vi "LogResult.vi"(5 "Mode":T1, 8 "Test Result":errorcluster, 10 "Test Artifact":T2 format="%x", 11 "VI Path":path) -> ()   [LabVIEW 2013]
uses:
  <vilib>/Heliosphere Research LLC/Advanced Plotting Toolkit/typedefs/PlotID.ctl
  ModeType.ctl
  OutputDirectory.vi
  <vilib>/Heliosphere Research LLC/Advanced Plotting Toolkit/Advanced Plotting Toolkit.lvlib
panel:
  out "Log To Disk":bool
  out "Status Out":string
  out "Picture":picture
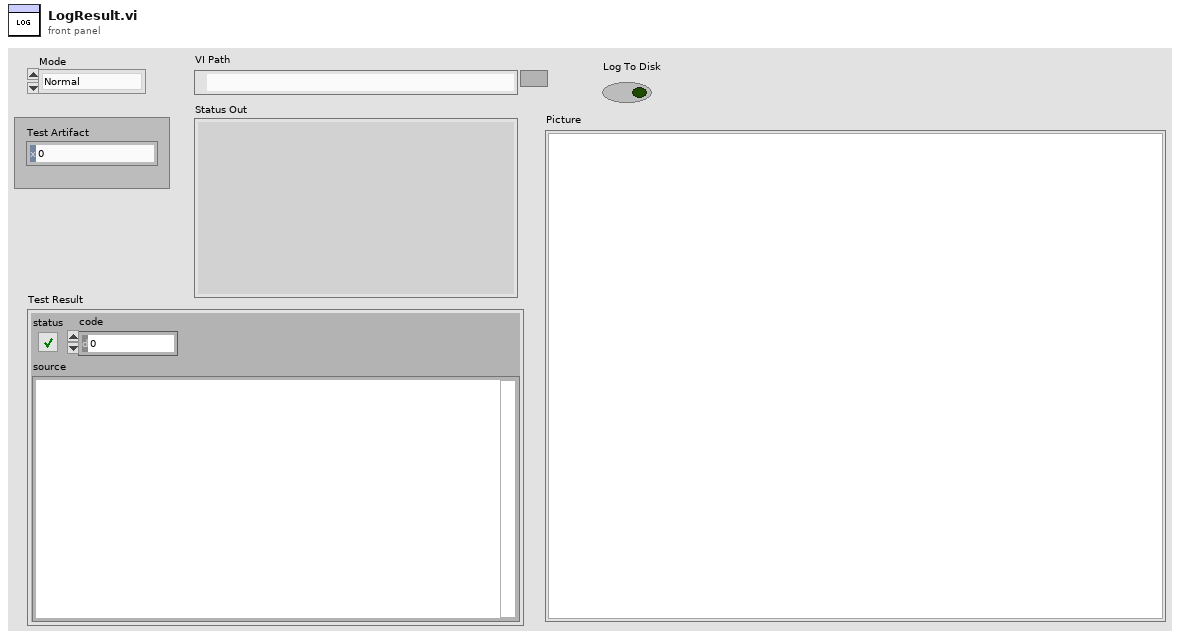
[diagram p1: front panel]
types:
  T1 = typedef "ModeType.ctl" = enum16{"Normal", "Expected Failure", "Skipped", "Broken"}
  T2 = typedef "Advanced Plotting Toolkit.lvlib/PlotID.ctl" = i32
  T3 = enum16{"open", "replace", "create", "open or create", "replace or create", "replace or create with confirmation"}
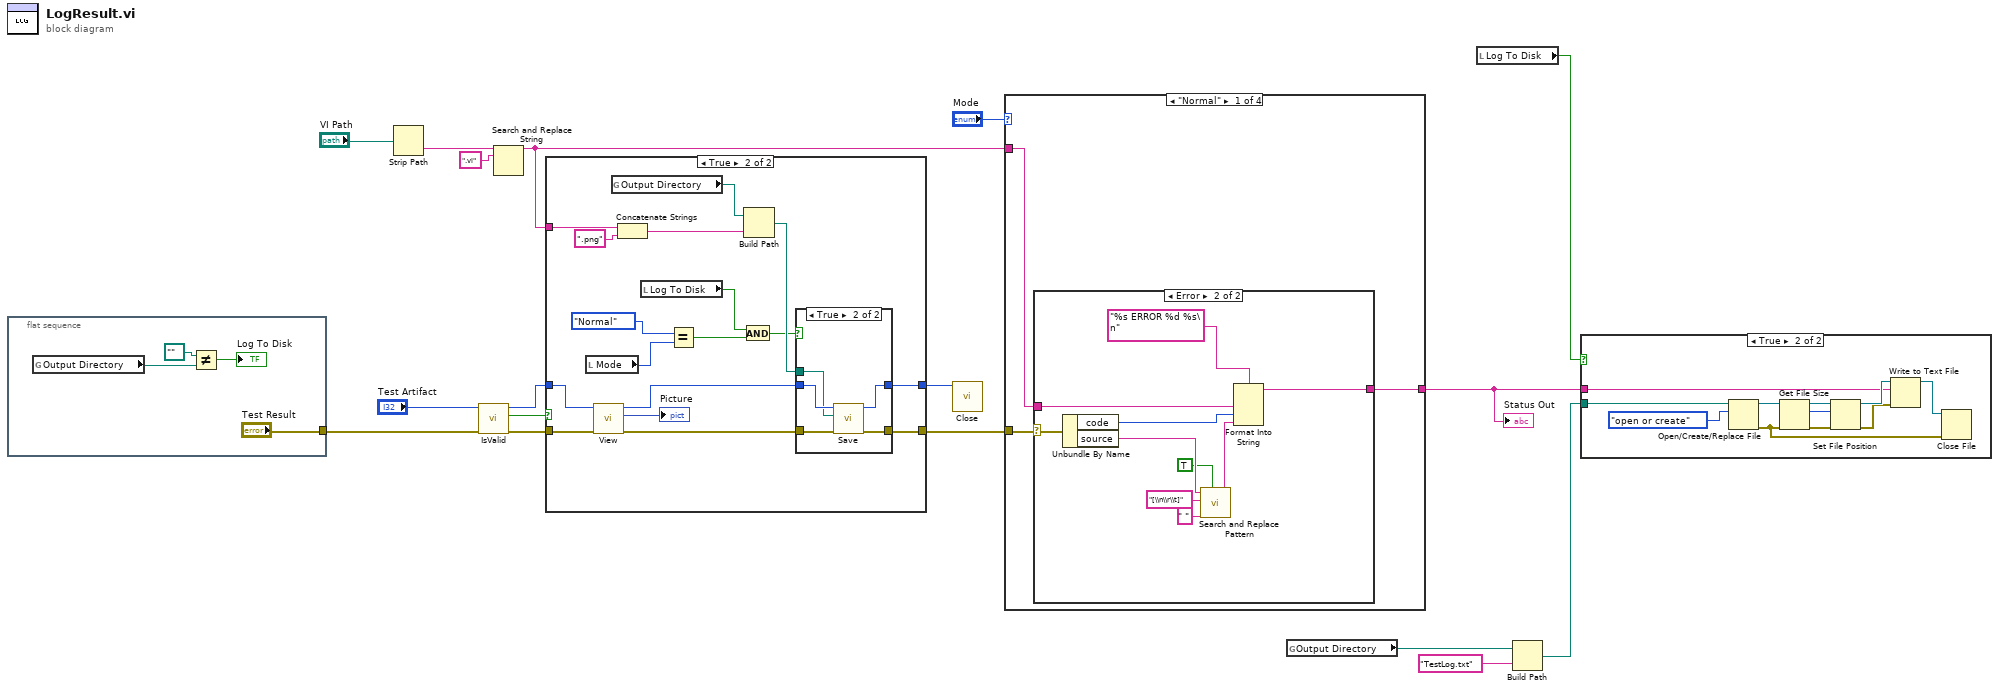
[diagram p0: block diagram]
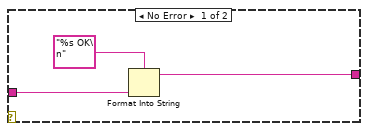
[diagram p2: hidden frame]
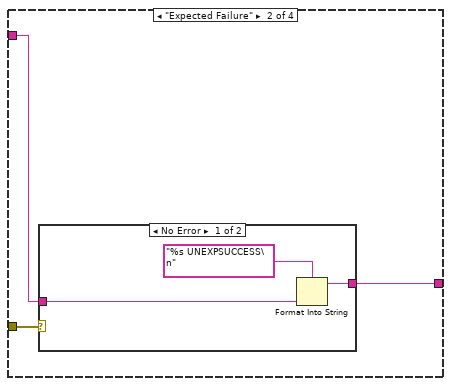
[diagram p3: hidden frame]
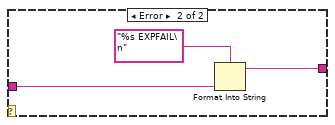
[diagram p4: hidden frame]
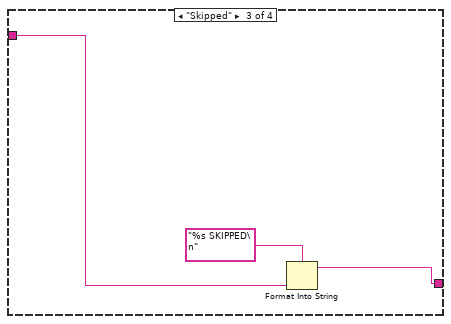
[diagram p5: hidden frame]
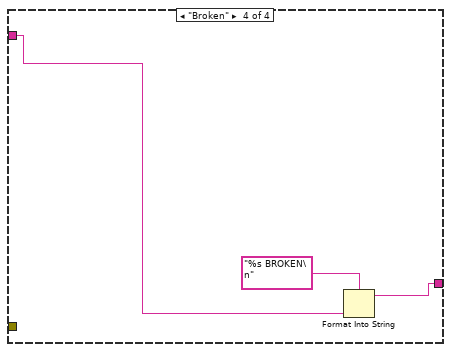
[diagram p6: hidden frame]
diagram:
  n1 = flat-sequence {
    tunnel: ["Test Result"] -> w4
    frame #0 {
      n2 = global read "OutputDirectory.vi" "Output Directory"() -> (w21:path)
      n3 = Not Equal?(x=path "" ("Output Directory"), y=w21) -> (x != y?=→"Log To Disk":bool)
    }
  }
  n4 = Strip Path(path="VI Path") -> (name=w11:string)  [unwired: 1 out]
  n5 = call <vilib>:"IsValid.vi"("error in (no error)"=w4, "Plot ID"="Test Artifact") -> ("error out"=w13:errorcluster, "Valid?"=w1:bool, "Plot ID Out"=w14:T2)  [unwired: 7 in]
  n6 = Search and Replace String(input string=w11, search string=".vi") -> (result string=w8:string)  [unwired: 6 in, 3 out]
  n7 = case shown="True" w1 {
    tunnel: w14 -> [w23 w40]
    tunnel: w13 -> [w22 w37]
    tunnel: w8 -> [_ w34]
    tunnel: [w23 w32] -> w7
    tunnel: [w22 w31] -> w5
    frame False {
    }
    frame True {
      n8 = local read "Mode"() -> (w29:T1)
      n9 = call <vilib>:"View.vi"("error in (no error)"=w37, "Plot ID"=w40) -> ("error out"=w39:errorcluster, "Picture"=→"Picture":picture, "Plot ID Out"=w38:T2)  [unwired: 7 in]
      n10 = global read "OutputDirectory.vi" "Output Directory"() -> (w25:path)
      n11 = Concatenate Strings(w34, ".png" ("string")) -> (w33:string)
      n12 = local read "Log To Disk"() -> (w27:bool)
      n13 = Equal?(x=ModeType."Normal" ("Mode"), y=w29) -> (x = y?=w28:bool)
      n14 = And(x=w27, y=w28) -> (x .and. y?=w26:bool)
      n15 = Build Path(base path=w25, name or relative path=w33) -> (appended path=w36:path)
      n16 = case shown="True" w26 {
        tunnel: w39 -> [w41 w47]
        tunnel: w38 -> [w42 w46]
        tunnel: w36 -> [_ w45]
        tunnel: [w42 w44] -> w32
        tunnel: [w41 w43] -> w31
        frame False {
        }
        frame True {
          n17 = call <vilib>:"Save.vi"("error in (no error)"=w47, "Path"=w45, "Plot ID In"=w46) -> ("error out"=w43:errorcluster, "Plot ID Out"=w44:T2)  [unwired: 7 in]
        }
      }
    }
  }
  n18 = call <vilib>:"Close.vi"("Plot ID"=w7) -> ()  [unwired: 10 in, 1 out]
  n19 = case shown="\"Normal\"" "Mode" {
    tunnel: [w50 w64 w73 w76] -> w9
    tunnel: w8 -> [w49 w65 w74 w77]
    tunnel: w5 -> [w48 w66 _ _]
    frame "Normal" {
      n20 = case shown="Error" w48 {
        selector: w48 -> [_ w63]
        tunnel: [w51 w61] -> w50
        tunnel: w49 -> [w52 w60]
        frame No Error {
          n21 = Format Into String(format string="%s OK\n", w52) -> (resulting string=w51:string)  [unwired: 2 in, 1 out]
        }
        frame Error {
          n22 = Unbundle By Name(w63) -> ("code"=w59:i32, "source"=w56:string)
          n23 = call <vilib>:"Search and Replace Pattern.vi"("string"=w56, "regular expression (\"\")"="[\\n\\r\\t]" ("regular expression (\"\")"), "replace string (\"\")"=" " ("replace string (\"\")"), "replace all? (F)"=TRUE) -> ("result string"=w55:string)  [unwired: 1 in, 1 out]
          n24 = Format Into String(format string="%s ERROR %d %s\n", w60, w59, w55) -> (resulting string=w61:string)  [unwired: 2 in, 1 out]
        }
      }
    }
    frame "Expected Failure" {
      n25 = case shown="No Error" w66 {
        tunnel: w65 -> [w68 w71]
        tunnel: [w67 w70] -> w64
        frame No Error {
          n26 = Format Into String(format string="%s UNEXPSUCCESS\n", w68) -> (resulting string=w67:string)  [unwired: 2 in, 1 out]
        }
        frame Error {
          n27 = Format Into String(format string="%s EXPFAIL\n", w71) -> (resulting string=w70:string)  [unwired: 2 in, 1 out]
        }
      }
    }
    frame "Skipped" {
      n28 = Format Into String(format string="%s SKIPPED\n", w74) -> (resulting string=w73:string)  [unwired: 2 in, 1 out]
    }
    frame "Broken" {
      n29 = Format Into String(format string="%s BROKEN\n", w77) -> (resulting string=w76:string)  [unwired: 2 in, 1 out]
    }
  }
  "Status Out" <- w9
  n30 = global read "OutputDirectory.vi" "Output Directory"() -> (w2:path)
  n31 = local read "Log To Disk"() -> (w3:bool)
  n32 = Build Path(base path=w2, name or relative path="TestLog.txt") -> (appended path=w16:path)
  n33 = case shown="True" w3 {
    tunnel: w16 -> [_ w89]
    tunnel: w9 -> [_ w79]
    frame False {
    }
    frame True {
      n34 = Open/Create/Replace File(file path (use dialog)=w89, operation (0:open)=T3."open or create") -> (refnum out=w87:refnum<file>, error out=w80:errorcluster)  [unwired: 4 in, 1 out]
      n35 = Get File Size(file=w87, error in=w80) -> (refnum out=w84:refnum<file>, size (in bytes)=w85:i64, 0:w86:errorcluster)
      n36 = Set File Position(offset (in bytes) (0)=w85, refnum=w84, error in=w86) -> (refnum out=w83:refnum<file>, error out=w82:errorcluster)  [unwired: 1 in]
      n37 = Write to Text File(file (use dialog)=w83, text=w79, error in=w82) -> (refnum out=w81:refnum<file>)  [unwired: 1 in, 2 out]
      n38 = Close File(refnum=w81, error in=w80) -> ()  [unwired: 2 out]
    }
  }
